vi "Convert dBV to Volts.vi"(4 "dBV":dbl format="%.2f") -> (1 "Volts":dbl format="%.2f")   [LabVIEW 2011]
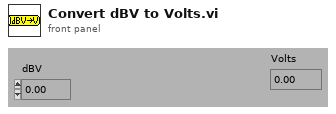
[diagram p1: front panel]
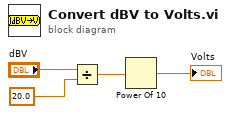
[diagram p0: block diagram]
diagram:
  n1 = Divide(x="dBV", y=20.0) -> (x/y=w3:dbl)
  n2 = Power Of 10(x=w3) -> (10^x=→"Volts":dbl)
